vi "Read Global Locked.vi"(7 "Semaphore Timeout":i32=-1, 8 "error in (no error)":errorcluster, 11 "GrabberWheels in":refnum<class "GrabberWheels.lvclass">) -> (0 "error out":errorcluster, 1 "Semaphore Timed Out":bool, 2 "Global":refnum<class "System.lvclass">, 3 "GrabberWheels out":refnum<class "GrabberWheels.lvclass">)   [LabVIEW 2013, in "GrabberWheels.lvclass"]
uses:
  GrabberWheels.lvclass
  System/System.lvclass
  Robot Global Data.vi
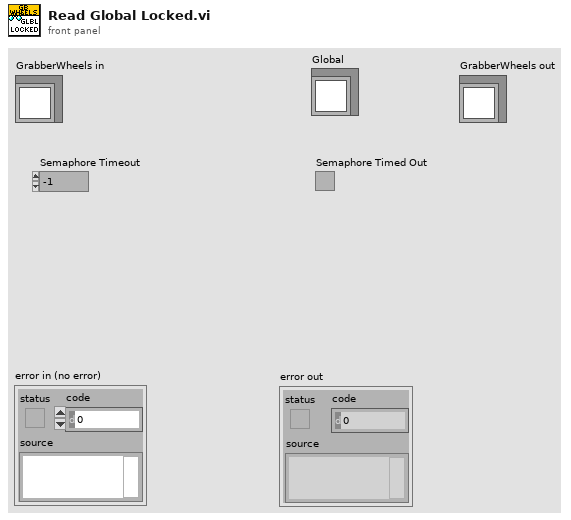
[diagram p1: front panel]
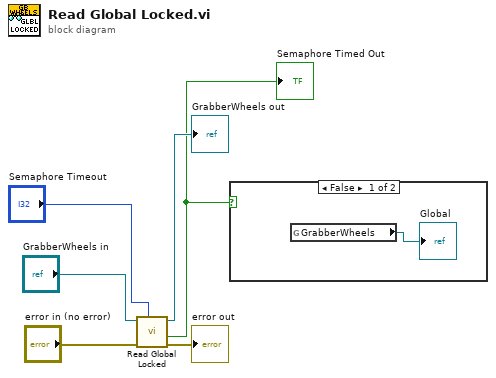
[diagram p0: block diagram]
diagram:
  n1 = call-parent "Read Global Locked.vi"("Semaphore Timeout"="Semaphore Timeout", "error in (no error)"="error in (no error)", "System in"="GrabberWheels in") -> ("error out"=→"error out":errorcluster, "Semaphore Timed Out"=w1:bool, "System out"=→"GrabberWheels out":refnum<class "GrabberWheels.lvclass">)  [unwired: 5 in, 1 out]
  "Semaphore Timed Out" <- w1
  n2 = case shown="False" w1 {
    frame False {
      n3 = global read "Robot Global Data.vi" "GrabberWheels"() -> (→"Global":refnum<class "GrabberWheels.lvclass">)
    }
    frame True {
    }
  }
